vi "LDT Telescope Loop.vi"(9 "topic":string="TCS.TCSSharedVariables.TCSHighLevelStatusSV.TCSTcsStatusSV", 10 "messageEvent":refnum<user-event>, 11 "ActiveMQBroker out":refnum<class "ActiveMQBroker.lvclass">) -> ()   [LabVIEW 2022 SP3, in "LDT Telescope.lvclass"]
uses:
  LDT Telescope.lvclass
  TCS/DCT-related/Common/Communication/ActiveMQ/ActiveMQBroker/ActiveMQBroker.lvclass
panel:
  in  "Tab Control":T1(tab)
  out "TCS Status":string
  out "AOS":string
  out "AOS data packet":string
  out "XML String":string
  out "Timestamp":timestamp
  in  "error in (no error)":errorcluster
  in  "stopReader":bool
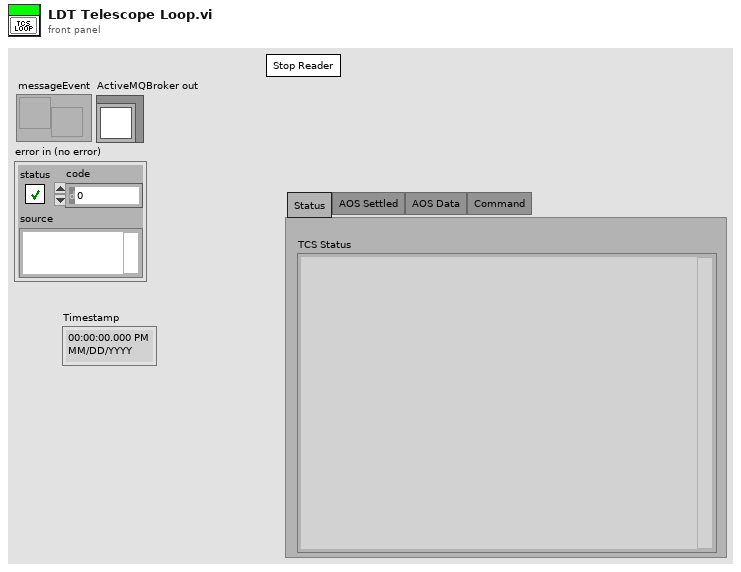
[diagram p1: front panel]
types:
  T1 = enum32{"Status", "AOS Settled", "AOS Data", "Command"}
  T2 = typedef "CC cluster Object.ctl" = cluster{"Object":cluster{"Name":string}, "Sidereal Rate":T3, "RA and DEC":T4, "Proper Motion":T5, "Offsets":T6, "Equinox":T7, "Parallax":T8, "Rotator":T9, "Frame":T10, "Frac Rate":dbl, "Wavelength":dbl}
  T3 = typedef "CC cluster sidereal rate.ctl" = cluster{"dRA":dbl, "dDEC":dbl}
  T4 = typedef "CC cluster RA and DEC.ctl" = cluster{"RA":dbl, "DEC":dbl}
  T5 = typedef "cc cluster muRA muDEC.ctl" = cluster{"muRA":dbl, "muDEC":dbl, "Epoch":dbl}
  T6 = typedef "CC cluster Telescope Offsets.ctl" = cluster{"xi":dbl, "eta":dbl, "Offset Type":enum16{"SIMPLE", "TPLANE", "PA"}}
  T7 = typedef "Telescope cluster Equinox.ctl" = cluster{"Equinox Year":i32, "Equinox Prefix":string}
  T8 = typedef "Telescope cluster Parallax.ctl" = cluster{"Parallax":dbl, "rv kps":dbl}
  T9 = typedef "Telescope cluster Rotator.ctl" = cluster{"Frame":enum16{"Target", "Fixed"}, "PA":dbl}
  T10 = typedef "Telesope ring Frame.ctl" = enum16{"FK4", "FK5", "APPT", "GAPPT", "AZEL"}
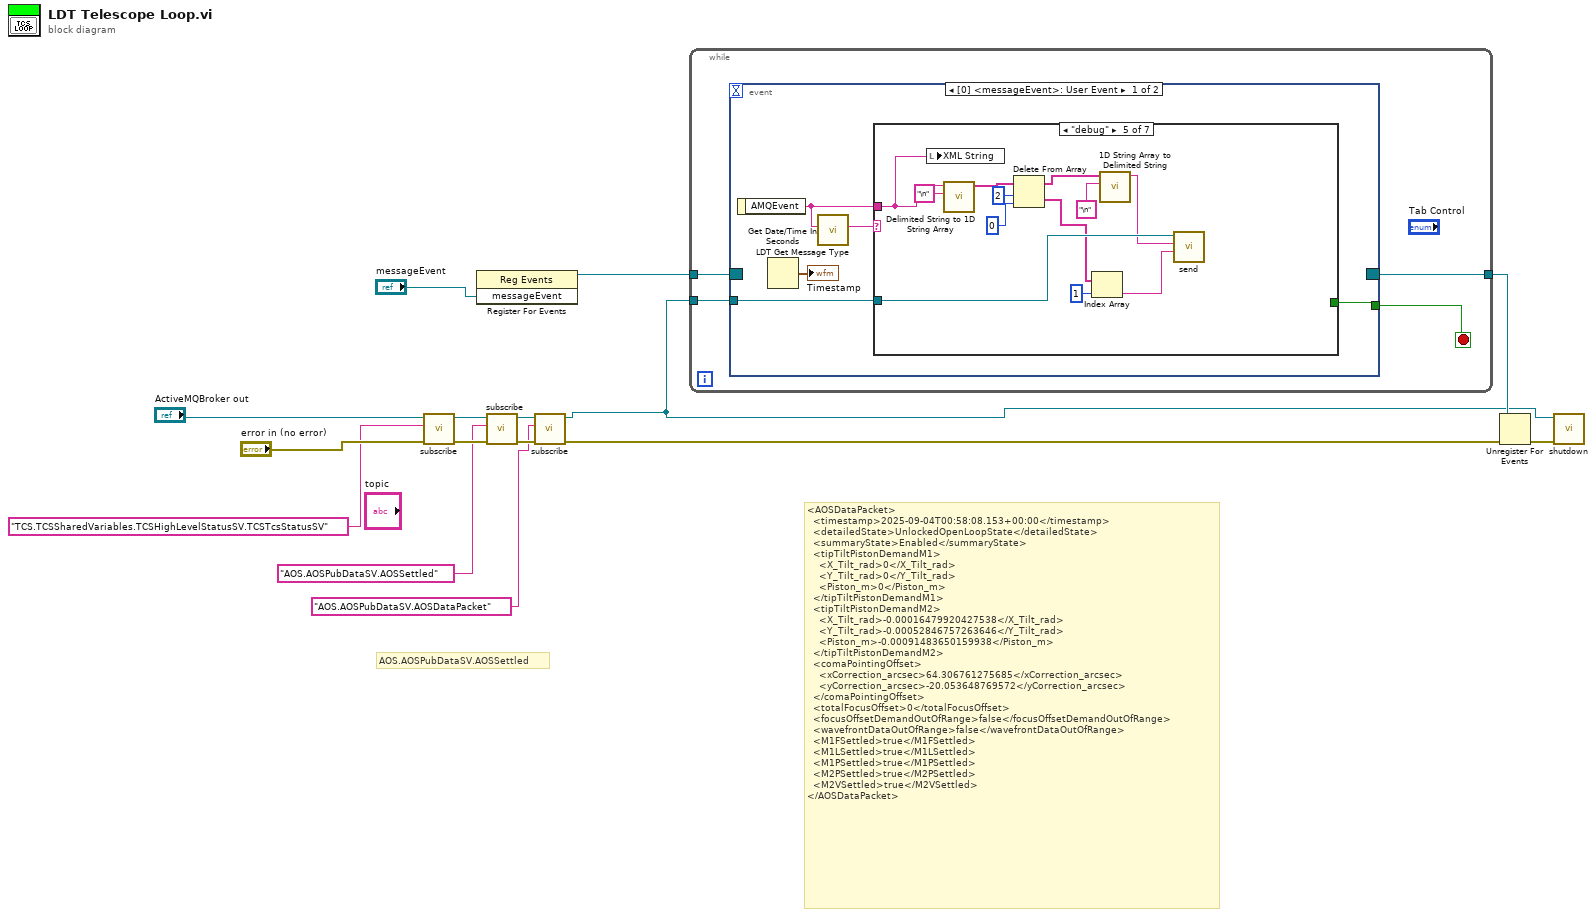
[diagram p0: block diagram]
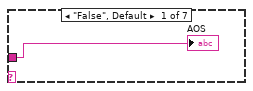
[diagram p2: hidden frame]
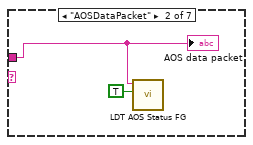
[diagram p3: hidden frame]
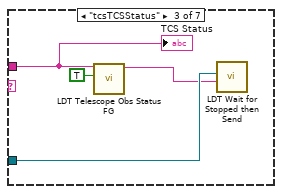
[diagram p4: hidden frame]
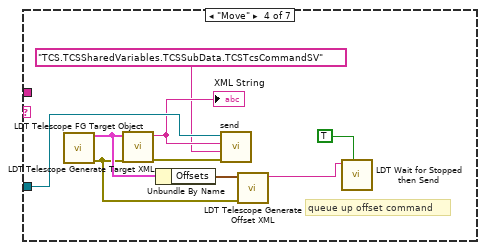
[diagram p5: hidden frame]
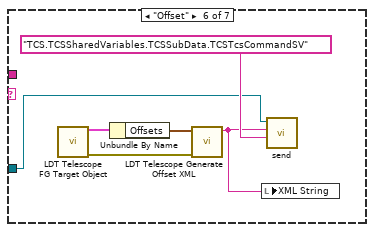
[diagram p6: hidden frame]
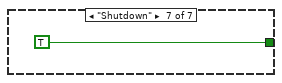
[diagram p7: hidden frame]
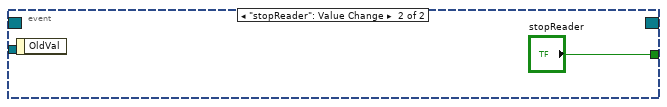
[diagram p8: hidden frame]
diagram:
  # "AOS.AOSPubDataSV.AOSSettled"
  # "<AOSDataPacket>\n  <timestamp>2025-09-04T00:58:08.153+00:00</timestamp>\n  <detailedState>UnlockedOpenLoopState</detailedState>\n  <summaryState>Enabled</summaryState>\n  <tipTiltPistonDemandM1>\n    <X_Tilt_rad>0</X_Tilt_rad>\n    <Y_Tilt_rad>0</Y_Tilt_rad>\n    <Piston_m>0</Piston_m>\n  </tipTiltPistonDemandM1>\n  <tipTiltPistonDemandM2>\n    <X_Tilt_rad>-0.00016479920427538</X_Tilt_rad>\n    <Y_Tilt_rad>-0.00052846757263646</Y_Tilt_rad>\n    <Piston_m>-0.00091483650159938</Piston_m>\n  </tipTiltPistonDemandM2>\n  <comaPointingOffset>\n    <xCorrection_arcsec>64.306761275685</xCorrection_arcsec>\n    <yCorrection_arcsec>-20.053648769572</yCorrection_arcsec>\n  </comaPointingOffset>\n  <totalFocusOffset>0</totalFocusOffset>\n  <focusOffsetDemandOutOfRange>false</focusOffsetDemandOutOfRange>\n  <wavefrontDataOutOfRange>false</wavefrontDataOutOfRange>\n  <M1FSettled>true</M1FSettled>\n  <M1LSettled>true</M1LSettled>\n  <M1PSettled>true</M1PSettled>\n  <M2PSettled>true</M2PSettled>\n  <M2VSettled>true</M2VSettled>\n</AOSDataPacket>"
  n1 = call-dynamic "subscribe.vi"("error in (no error)"="error in (no error)", "source"="TCS.TCSSharedVariables.TCSHighLevelStatusSV.TCSTcsStatusSV", "ActiveMQBroker in"="ActiveMQBroker out") -> ("error out"=w8:errorcluster, "ActiveMQBroker out"=w9:refnum<class "ActiveMQBroker.lvclass">)  [unwired: 7 in]
  n2 = register-events("messageEvent") -> (reference out=w15:refnum<event-registration>)  [unwired: 2 in, 1 out]
  n3 = call-dynamic "subscribe.vi"("error in (no error)"=w8, "source"="AOS.AOSPubDataSV.AOSSettled", "ActiveMQBroker in"=w9) -> ("error out"=w4:errorcluster, "ActiveMQBroker out"=w6:refnum<class "ActiveMQBroker.lvclass">)  [unwired: 7 in]
  n4 = call-dynamic "subscribe.vi"("error in (no error)"=w4, "source"="AOS.AOSPubDataSV.AOSDataPacket", "ActiveMQBroker in"=w6) -> ("error out"=w3:errorcluster, "ActiveMQBroker out"=w5:refnum<class "ActiveMQBroker.lvclass">)  [unwired: 7 in]
  n5 = while {
    tunnel: w15 -> [w19]
    tunnel: [w18] -> w14
    tunnel: w5 -> [w16]
    stop <- w17 stop-if-true
    n6 = event shown="[0] <messageEvent>: User Event" {
      selector: w19 -> [_ _]
      dyn-events: [_ _] -> w18
      timeout: _ -> [_ _]
      tunnel: [w24 "stopReader"] -> w17
      tunnel: w16 -> [w23 _]
      event User Event {
        n7 = event-data() -> ("AMQEvent"=w21:string)  [unwired: 1 in]
        n8 = Get Date/Time In Seconds() -> (seconds since 1Jan1904=→"Timestamp":timestamp)
        n9 = call "LDT Get Message Type.vi"("String"=w21) -> ("submatch 1"=w20:string)  [unwired: 10 in]
        n10 = case shown="\"debug\"" w20 {
          tunnel: w21 -> [w25 w27 w28 _ w41 _ _]
          tunnel: [_ _ _ _ _ _ TRUE] -> w24
          tunnel: w23 -> [_ _ w30 w40 w52 w56 _]
          frame "False", Default {
            "AOS" <- w25
          }
          frame "AOSDataPacket" {
            n11 = call "LDT AOS Status FG.vi"("Write?"=TRUE, "AOS String"=w27) -> ()  [unwired: 8 in, 2 out]
            "AOS data packet" <- w27
          }
          frame "tcsTCSStatus" {
            n12 = call "LDT Telescope Obs Status FG.vi"("Write?"=TRUE, "String"=w28) -> ("status string out"=w29:string)  [unwired: 8 in, 1 out]
            n13 = call "LDT Wait for Stopped then Send.vi"("XML Status"=w29, "ActiveMQBroker in"=w30) -> ()  [unwired: 9 in, 1 out]
            "TCS Status" <- w28
          }
          frame "Move" {
            # "queue up offset command"
            n14 = call "LDT Telescope FG Target Object.vi"() -> ("error out"=w35:errorcluster, "Object out"=w36:T2)  [unwired: 10 in]
            n15 = call "LDT Telescope Generate Target XML.vi"("error in (no error)"=w35, "Object out"=w36) -> ("error out"=w38:errorcluster, "XML String"=w39:string)  [unwired: 8 in]
            "XML String" <- w39
            n16 = Unbundle By Name(w36) -> ("Offsets"=w37:T6)
            n17 = call-dynamic "send.vi"("error in (no error)"=w38, "topic"="TCS.TCSSharedVariables.TCSSubData.TCSTcsCommandSV", "message"=w39, "ActiveMQBroker in"=w40) -> ()  [unwired: 6 in, 2 out]
            n18 = call "LDT Telescope Generate Offset XML.vi"("error in"=w35, "Offsets"=w37) -> ("XML String"=w32:string)  [unwired: 9 in]
            n19 = call "LDT Wait for Stopped then Send.vi"("add to q"=TRUE, "msg to send"=w32) -> ()  [unwired: 9 in, 1 out]
          }
          frame "debug" {
            n20 = local write "XML String"(w41) -> ()
            n21 = call <vilib>:"Delimited String to 1D String Array.vi"("delimiter"="\n", "delimited string"=w41) -> ("string array"=w50:string[])  [unwired: 9 in]
            n22 = Delete From Array(array=w50, length=2, index=0) -> (deleted portion=w42:string[], array with subset deleted=w43:string[])
            n23 = Index Array(array=w42, index=1) -> (element=w44:string)
            n24 = call <vilib>:"1D String Array to Delimited String.vi"("delimiter"="\n", "string array"=w43) -> ("delimited string"=w46:string)  [unwired: 9 in]
            n25 = call-dynamic "send.vi"("topic"=w44, "message"=w46, "ActiveMQBroker in"=w52) -> ()  [unwired: 7 in, 2 out]
          }
          frame "Offset" {
            n26 = call "LDT Telescope FG Target Object.vi"() -> ("error out"=w55:errorcluster, "Object out"=w58:T2)  [unwired: 10 in]
            n27 = Unbundle By Name(w58) -> ("Offsets"=w53:T6)
            n28 = call "LDT Telescope Generate Offset XML.vi"("error in"=w55, "Offsets"=w53) -> ("XML String"=w54:string)  [unwired: 9 in]
            n29 = local write "XML String"(w54) -> ()
            n30 = call-dynamic "send.vi"("topic"="TCS.TCSSharedVariables.TCSSubData.TCSTcsCommandSV", "message"=w54, "ActiveMQBroker in"=w56) -> ()  [unwired: 7 in, 2 out]
          }
          frame "Shutdown" {
          }
        }
      }
      event "stopReader": Value Change {
        n31 = event-data() -> ()  [unwired: 1 in, 1 out]
      }
    }
  }
  n32 = Unregister For Events(event registration refnum=w14, error in=w3) -> (error out=w10:errorcluster)
  n33 = call-dynamic "shutdown.vi"("error in (no error)"=w10, "ActiveMQBroker in"=w5) -> ()  [unwired: 8 in, 2 out]
